vi "Init Events.vi"(8 "error in (no error)":errorcluster, 11 "MuxPanel in":refnum<class "MuxPanel.lvclass">) -> (0 "error out":errorcluster, 3 "MuxPanel out":refnum<class "MuxPanel.lvclass">)   [LabVIEW 2022 SP3, in "TouchControl.lvlib" / "MuxPanel.lvclass"]
uses:
  MuxPanel.lvclass
  MuxPanel.lvclass/MuxPanel.ctl
  Connection.ctl
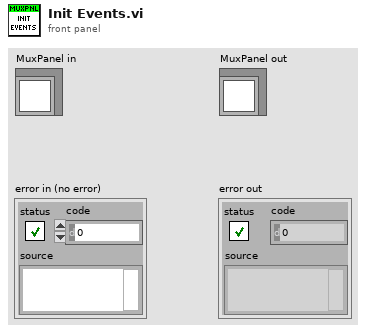
[diagram p1: front panel]
types:
  T1 = typedef "TouchControl.lvlib/MuxPanel.lvclass/Connection.ctl" = cluster{"Mux Index":i32, "Input":i32, "Output":i32}
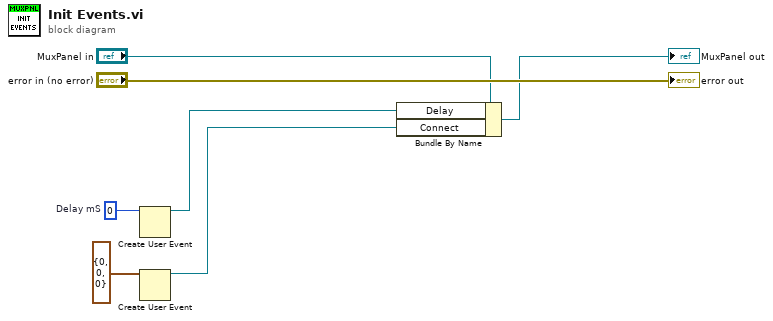
[diagram p0: block diagram]
diagram:
  w6 = 0  # Delay mS
  n1 = Create User Event(user event datatype=w6) -> (user event=w5:refnum<user-event>)  [unwired: 1 in, 1 out]
  n2 = Create User Event(user event datatype=T1 {"Mux Index"=0, "Input"=0, "Output"=0} ("Connection")) -> (user event=w1:refnum<user-event>)  [unwired: 1 in, 1 out]
  n3 = Bundle By Name(cluster="MuxPanel in", "Delay"=w5, "Connect"=w1) -> (→"MuxPanel out":refnum<class "MuxPanel.lvclass">)
  "error out" <- "error in (no error)"
